vi "GetRoot.vi"(0 "object in":refnum<class "Tree.lvclass">, 5 "Error In":errorcluster) -> (14 "object out":refnum<class "Tree.lvclass">, 15 "Root":refnum<class "Node.lvclass">, 19 "Error Out":errorcluster)   [LabVIEW 2024, in "Tree.lvclass"]
uses:
  <resource>/Framework/Providers/Open_GDS/ClassProviders/Provider_LvNativeClass/Templates/NativeBaseTemplate/NativeBaseTemplate.lvclass/NativeBaseTemplate.ctl
  Tree.lvclass
  Tree.lvclass/Tree.ctl
  Node_class/Node.lvclass
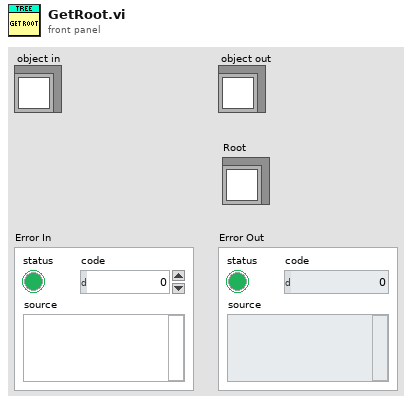
[diagram p1: front panel]
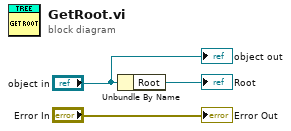
[diagram p0: block diagram]
diagram:
  n1 = Unbundle By Name("object in") -> ("Root"=→"Root":refnum<class "Node.lvclass">)
  "Error Out" <- "Error In"
  "object out" <- "object in"
